vi "number_split.vi"(1 "Numeric":dbl format="%#_13g") -> (0 "Split Numbers":dbl[](array[numeric]))   [LabVIEW 2020]
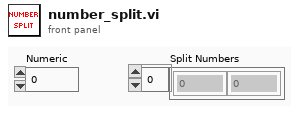
[diagram p1: front panel]
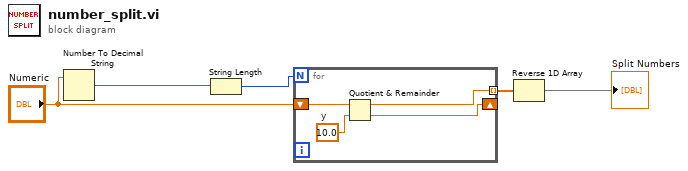
[diagram p0: block diagram]
diagram:
  n1 = Number To Decimal String(number="Numeric") -> (decimal integer string=w1:string)  [unwired: 1 in]
  n2 = String Length(string=w1) -> (length=w2:i32)
  n3 = for {
    N: w2 -> [_]
    shift-right: [w6] -> _
    shift-left: "Numeric" -> [w9]
    tunnel: [w7] -> w4 mode=indexing
    w8 = 10.0  # y
    n4 = Quotient & Remainder(x=w9, y=w8) -> (x-y*floor(x/y)=w7:dbl, floor(x/y)=w6:dbl)
  }
  n5 = Reverse 1D Array(array=w4) -> (reversed array=→"Split Numbers":dbl[])
